vi "COMTRADE Read Private Inf (N Entries).vi"(7 "entry names":string[](array[string]), 8 "error in (no error)":errorcluster, 9 "section name":string, 10 "manufacturer name":string, 11 "task in":T1={"file refnums"=[], "Data Object"=refnum, "config info"={"station_name"="", "rec_dev_id"="", "rev_year"=1999.0, "TT"=0, "##A"=0, "##D"=0, "analog channel info"=[], "status channel info"=[], "lf"=50.0, "nrates"=0, "samp info"=[], "initial timestamp"=timestamp(0 s since 1904-01-01), "trigger timestamp"=timestamp(0 s since 1904-01-01), "ft"=enum."Binary", "timemult"=1.0}, "public inf content"={"Source"="", "Record Type"=enum."Unknown", "Phase ID"="", "Event Description"="", "Device ID"="", "Distance of Fault"=-1.0, "Distance Unit"=enum."Miles", "Max_Current"=inf, "Min_Current"=-inf, "Max_Voltage"=inf, "Min_Voltage"=-inf, "EventNoteCount"=0, "Event Information"=[]}, "private inf content"=[], "internal buffers"={"start index"=1, "config to public inf"=enum."disabled", "static config info"="", "static file_des record inf"="", "static file_des channel inf"="", "public inf"="", "private inf"=""}} {"public inf content"."Event Information"."min sample number" max=9999999999; "public inf content"."Event Information"."max sample number" max=9999999999; "config info"."nrates" max=999; "config info"."status channel info"."Dn" min=1 max=999999; "config info"."analog channel info"."An" min=1 max=999999; "config info"."trigger timestamp" format="%<%H:%M:%S%6u\n%d/%m/%Y>T"; "config info"."initial timestamp" format="%<%H:%M:%S%6u\n%d/%m/%Y>T"; "config info"."##D" max=999999; "config info"."##A" max=999999; "config info"."TT" min=1 max=999999; "config info"."rev_year" min=1999.0 max=1999.0}) -> (0 "error out":errorcluster, 1 "entry values":string[](array[string]), 3 "task out":T1={"file refnums"=[], "Data Object"=refnum, "config info"={"station_name"="", "rec_dev_id"="", "rev_year"=1999.0, "TT"=0, "##A"=0, "##D"=0, "analog channel info"=[], "status channel info"=[], "lf"=50.0, "nrates"=0, "samp info"=[], "initial timestamp"=timestamp(0 s since 1904-01-01), "trigger timestamp"=timestamp(0 s since 1904-01-01), "ft"=enum."Binary", "timemult"=1.0}, "public inf content"={"Source"="", "Record Type"=enum."Unknown", "Phase ID"="", "Event Description"="", "Device ID"="", "Distance of Fault"=-1.0, "Distance Unit"=enum."Miles", "Max_Current"=inf, "Min_Current"=-inf, "Max_Voltage"=inf, "Min_Voltage"=-inf, "EventNoteCount"=0, "Event Information"=[]}, "private inf content"=[], "internal buffers"={"start index"=1, "config to public inf"=enum."disabled", "static config info"="", "static file_des record inf"="", "static file_des channel inf"="", "public inf"="", "private inf"=""}} {"public inf content"."Event Information"."min sample number" max=9999999999; "public inf content"."Event Information"."max sample number" max=9999999999; "config info"."nrates" max=999; "config info"."status channel info"."Dn" min=1 max=999999; "config info"."analog channel info"."An" min=1 max=999999; "config info"."trigger timestamp" format="%<%H:%M:%S%6u\n%d/%m/%Y>T"; "config info"."initial timestamp" format="%<%H:%M:%S%6u\n%d/%m/%Y>T"; "config info"."##D" max=999999; "config info"."##A" max=999999; "config info"."TT" min=1 max=999999; "config info"."rev_year" min=1999.0 max=1999.0}, 4 "entries found?":bool[](array[boolean]))   [LabVIEW 2013, in "NI_EP_COMTRADE.lvlib"]
doc: "Reads information from the private sections of the optionally specified .inf file. You must set <B>open mode</B> to Open (read only) in the COMTRADE Open VI to open the .inf file. Otherwise this VI returns an error."
uses:
  <vilib>/addons/Electrical Power/File IO/NI_EP_COMTRADE.lvlib
  <vilib>/addons/Electrical Power/File IO/COMTRADE/typedefs/ep_Task.ctl
  <vilib>/addons/Electrical Power/File IO/COMTRADE/typedefs/ep_Config Info.ctl
  <vilib>/addons/Electrical Power/File IO/COMTRADE/typedefs/ep_Analog Channel Info.ctl
  <vilib>/addons/Electrical Power/File IO/COMTRADE/typedefs/ep_Status Channel Info.ctl
  <vilib>/addons/Electrical Power/File IO/COMTRADE/typedefs/ep_File Format.ctl
  <vilib>/addons/Electrical Power/File IO/COMTRADE/typedefs/ep_Public Inf Content.ctl
  <vilib>/addons/Electrical Power/File IO/COMTRADE/typedefs/ep_Public Event Inf.ctl
  <vilib>/addons/Electrical Power/File IO/COMTRADE/typedefs/ep_Private Inf Content.ctl
  <vilib>/Platform/storage/Storage.llb/Get Property (Storage Refnums).vi
  <vilib>/Platform/storage/Storage.llb/Get Property (I32).vi
  <vilib>/Platform/storage/Storage.llb/Get Property (String).vi
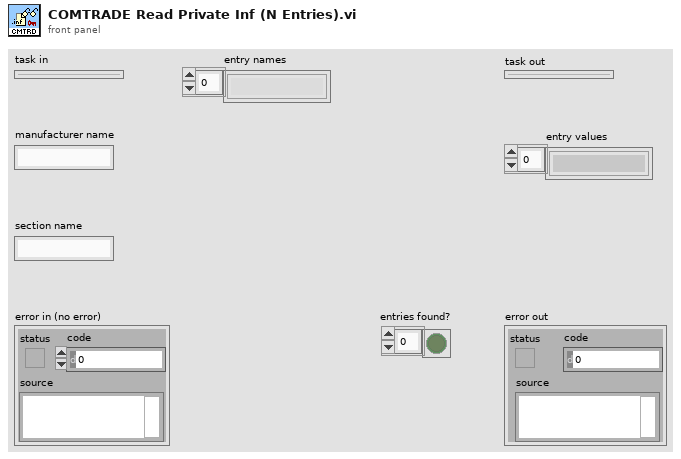
[diagram p1: front panel]
types:
  T1 = typedef "NI_EP_COMTRADE.lvlib/ep_Task.ctl" = cluster{"file refnums":refnum<file>[], "Data Object":refnum<k20>, "config info":T2, "public inf content":T6, "private inf content":T8, "internal buffers":cluster{"start index":u32, "config to public inf":enum16{"disabled", "enabled", "buffered"}, "static config info":string, "static file_des record inf":string, "static file_des channel inf":string, "public inf":string, "private inf":string}}
  T2 = typedef "NI_EP_COMTRADE.lvlib/ep_Config Info.ctl" = cluster{"station_name":string, "rec_dev_id":string, "rev_year":dbl, "TT":u32, "##A":u32, "##D":u32, "analog channel info":T3[], "status channel info":T4[], "lf":sgl, "nrates":u16, "samp info":cluster{"samp":sgl, "endsamp":u32}[], "initial timestamp":timestamp, "trigger timestamp":timestamp, "ft":T5, "timemult":sgl}
  T3 = typedef "NI_EP_COMTRADE.lvlib/ep_Analog Channel Info.ctl" = cluster{"An":u32, "ch_id":string, "ph":string, "ccbm":string, "uu":string, "a":sgl, "b":sgl, "skew":sgl, "min":i32, "max":i32, "primary":sgl, "secondary":sgl, "PS":enum16{"P", "S"}}
  T4 = typedef "NI_EP_COMTRADE.lvlib/ep_Status Channel Info.ctl" = cluster{"Dn":u32, "ch_id":string, "ph":string, "ccbm":string, "Y":bool}
  T5 = typedef "NI_EP_COMTRADE.lvlib/ep_File Format.ctl" = enum16{"ASCII", "Binary"}
  T6 = typedef "NI_EP_COMTRADE.lvlib/ep_Public Inf Content.ctl" = cluster{"Source":string, "Record Type":enum16{"Fault", "Unknown", "Misoperation", "Close", "Trip", "Reclose", "Power swing", "Simulation"}, "Phase ID":string, "Event Description":string, "Device ID":string, "Distance of Fault":dbl, "Distance Unit":enum16{"Miles", "Kilometers", "Percent of line", "Percent of setting", "Ohms"}, "Max_Current":dbl, "Min_Current":dbl, "Max_Voltage":dbl, "Min_Voltage":dbl, "EventNoteCount":u32, "Event Information":T7[]}
  T7 = typedef "NI_EP_COMTRADE.lvlib/ep_Public Event Inf.ctl" = cluster{"channel number":u32, "max value":dbl, "min value":dbl, "max sample number":u64, "min sample number":u64, "max sample text":string[], "min sample text":string[]}
  T8 = typedef "NI_EP_COMTRADE.lvlib/ep_Private Inf Content.ctl" = cluster{"Section Header":string, "Entry Names":string[], "Entry Values":string[]}[]
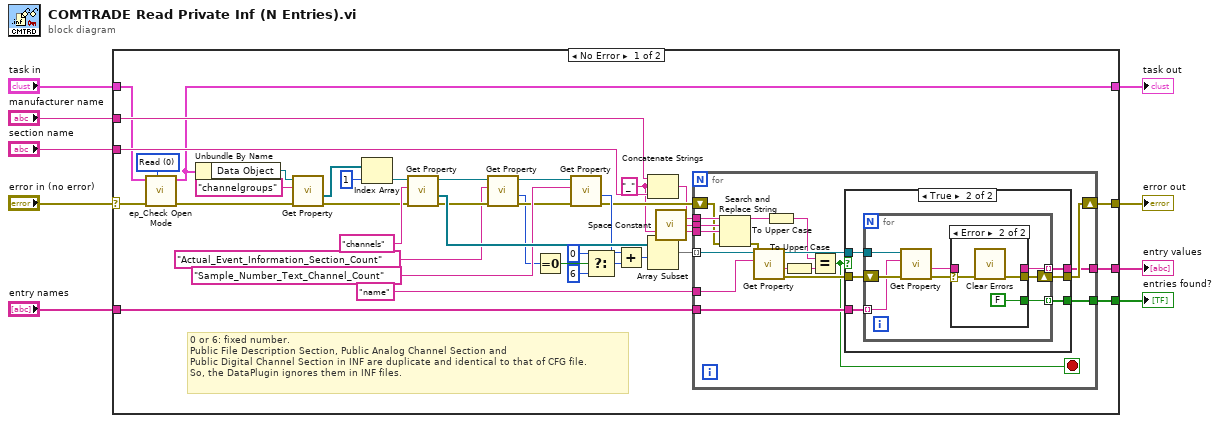
[diagram p0: block diagram]
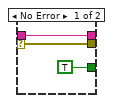
[diagram p3: hidden frame]
diagram:
  n1 = case shown="No Error" "error in (no error)" {
    selector: "error in (no error)" -> [w13 w87]
    tunnel: "task in" -> [w11 w88]
    tunnel: [w10 w88] -> w2
    tunnel: [w29 w87] -> w8
    tunnel: "manufacturer name" -> [w18 _]
    tunnel: "section name" -> [w33 _]
    tunnel: "entry names" -> [w31 _]
    tunnel: [w30 _] -> w4
    tunnel: [w15 _] -> w1
    frame No Error {
      w14 = u16 0 items=["Read", "Write"] ("file type")
      w16 = "_" ("string")
      # "0 or 6: fixed number.\nPublic File Description Section, Public Analog Channel Section and \nPublic Digital Channel Section in INF are duplicate and identical to that of CFG file. \nSo, the DataPlugin ignores them in INF files."
      n2 = call <vilib>:"ep_Check Open Mode.vi"("expected mode"=w14, "error in (no error)"=w13, "task in"=w11) -> ("error out"=w12:errorcluster, "task out"=w10:T1)  [unwired: 7 in]
      n3 = Unbundle By Name(w10) -> ("Data Object"=w47:refnum<k20>)
      n4 = call-poly <vilib>:"Get Property.vi"("error in (no error)"=w12, "Property name"="channelgroups", "storage refnum"=w47) -> ("error out"=w37:errorcluster, "Value"=w46:refnum<k20>[])  [unwired: 6 in, 1 out]
      n5 = Index Array(array=w46, index=1) -> (element=w42:refnum<k20>)
      n6 = call-poly <vilib>:"Get Property.vi"("error in (no error)"=w37, "Property name"="channels", "storage refnum"=w42) -> ("error out"=w28:errorcluster, "Value"=w41:refnum<k20>[], "storage refnum out"=w20:refnum<k20>)  [unwired: 6 in]
      n7 = call-poly <vilib>:"Get Property.vi"("error in (no error)"=w28, "Property name"="Actual_Event_Information_Section_Count", "storage refnum"=w20) -> ("error out"=w27:errorcluster, "Value"=w24:i32, "storage refnum out"=w19:refnum<k20>)  [unwired: 6 in]
      n8 = Equal To 0?(x=w24) -> (x = 0?=w25:bool)
      n9 = call-poly <vilib>:"Get Property.vi"("error in (no error)"=w27, "Property name"="Sample_Number_Text_Channel_Count", "storage refnum"=w19) -> ("error out"=w34:errorcluster, "Value"=w39:i32)  [unwired: 6 in, 1 out]
      n10 = Select(t=0 ("index"), s=w25, f=6 ("index")) -> (s? t:f=w23:i32)
      n11 = Add(x=w39, y=w23) -> (x+y=w40:i32)
      n12 = Concatenate Strings(w18, w16, w33) -> (w32:string)
      n13 = Array Subset(array=w41, index=w40) -> (w36:refnum<k20>[])  [unwired: 1 in]
      n14 = call <vilib>:"Space Constant.vi"() -> ("String"=w17:string)
      n15 = for {
        tunnel: w36 -> [w65] mode=indexing
        tunnel: "name" ("Property name") -> [w64]
        shift-right: [w59] -> w29
        shift-left: w34 -> [w53]
        tunnel: w32 -> [w56]
        tunnel: w31 -> [w62]
        tunnel: [w58] -> w30
        tunnel: w17 -> [w55]
        tunnel: w16 -> [w54]
        tunnel: [w50] -> w15
        stop <- w57 stop-if-true
        n16 = Search and Replace String(input string=w56, search string=w55, replace string=w54, error in=w53) -> (result string=w51:string, error out=w52:errorcluster)  [unwired: 4 in, 2 out]
        n17 = call-poly <vilib>:"Get Property.vi"("error in (no error)"=w52, "Property name"=w64, "storage refnum"=w65) -> ("error out"=w60:errorcluster, "Value"=w63:string, "storage refnum out"=w61:refnum<k20>)  [unwired: 6 in]
        n18 = To Upper Case(1:w51) -> (0:w49:string)
        n19 = To Upper Case(1:w63) -> (0:w48:string)
        n20 = Equal?(x=w49, y=w48) -> (x = y?=w57:bool)
        n21 = case shown="True" w57 {
          tunnel: w62 -> [_ w72]
          tunnel: w61 -> [_ w71]
          tunnel: w60 -> [w66 w70]
          tunnel: [_ w69] -> w58
          tunnel: [w66 w68] -> w59
          tunnel: [_ w67] -> w50
          frame False {
          }
          frame True {
            n22 = for {
              tunnel: w72 -> [w78] mode=indexing
              tunnel: w71 -> [w80]
              shift-right: [w74] -> w68
              shift-left: w70 -> [w79]
              tunnel: [w75] -> w69 mode=indexing
              tunnel: [w73] -> w67 mode=indexing
              n23 = call-poly <vilib>:"Get Property.vi"("error in (no error)"=w79, "Property name"=w78, "storage refnum"=w80) -> ("error out"=w77:errorcluster, "Value"=w76:string)  [unwired: 6 in, 1 out]
              n24 = case shown="Error" w77 {
                selector: w77 -> [w82 w86]
                tunnel: w76 -> [w83 _]
                tunnel: [w83 _] -> w75
                tunnel: [w82 w85] -> w74
                tunnel: [TRUE FALSE] -> w73
                frame No Error {
                }
                frame Error {
                  n25 = call <vilib>:"Clear Errors.vi"("error in (no error)"=w86) -> ("error out"=w85:errorcluster)  [unwired: 6 in]
                }
              }
            }
          }
        }
      }
    }
    frame Error {
    }
  }
  "error out" <- w8
  "entry values" <- w4
  "entries found?" <- w1
  "task out" <- w2
